vi "Turn_IMU.vi"(0 "Timeout (s)":dbl, 1 "Acceptable Error (Degrees)":dbl, 2 "Target (Degrees)":dbl) -> ()   [LabVIEW 2020]
uses:
  <vilib>/Rock Robotics/WPI/ThirdParty/REV Robotics/REVLib/Typedef/Spark MAX Control Type.ctl
  <vilib>/Rock Robotics/WPI/ThirdParty/Phoenix-LabVIEW/Pigeon IMU/CTRE_PigeonIMU_GetYPR.vi
panel:
  out "Times Target Successful":dbl
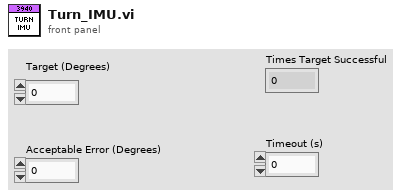
[diagram p1: front panel]
types:
  T1 = typedef "CTRE_PigeonIMU_DeviceRef.ctl" = cluster{"DeviceStatus":errorcluster, "Device Number":u8, "Type":T2, "Device ID":u32, "Handle":u64, "UsageFrame":u32, "Library Path":path}
  T2 = typedef "CTRE_PigeonIMU_ConnectionType.ctl" = u32
  T3 = typedef "WPI_MotorControlDeviceRef.ctl" = cluster{"DeviceStatus":errorcluster, "Type":T4, "PWM":cluster{"PWM Channel":T5, "DeadBand":T6}, "CAN":cluster{"Device Number":u8, "SetOutput VI Ref":variant, "GetOutput VI Ref":variant, "Enable VI Ref":variant, "Disable VI Ref":variant, "Data":variant}, "Invert":bool, "DIO PWM":cluster{"PWM \"Enable\" Channel":T5, "DIOChannel":T7, "PWM Rate":dbl}}
  T4 = typedef "WPI_MotorControlType.ctl" = enum16{"PWM", "CAN", "DIO PWM"}
  T5 = typedef "FPGA_DIOPWMChannel.ctl" = enum8{"PWM 0", "PWM 1", "PWM 2", "PWM 3", "PWM 4", "PWM 5", "PWM 6", "PWM 7", "PWM 8", "PWM 9", "PWM MXP 0", "PWM MXP 1", "PWM MXP 2", "PWM MXP 3", "PWM MXP 4", "PWM MXP 5", "PWM MXP 6", "PWM MXP 7", "PWM MXP 8", "PWM MXP 9", "Invalid"}
  T6 = typedef "WPI_PWMDeadband.ctl" = cluster{"Name":string, "maxPositivePwm":i32, "minPositivePwm":i32, "centerPwm":i32, "maxNegativePwm":i32, "minNegativePwm":i32, "angularRange":u16}
  T7 = typedef "FPGA_DIOChannel.ctl" = enum8{"DIO 0", "DIO 1", "DIO 2", "DIO 3", "DIO 4", "DIO 5", "DIO 6", "DIO 7", "DIO 8", "DIO 9", "DIO MXP 0", "DIO MXP 1", "DIO MXP 2", "DIO MXP 3", "DIO MXP 4", "DIO MXP 5", "DIO MXP 6", "DIO MXP 7", "DIO MXP 8", "DIO MXP 9", "DIO MXP 10", "DIO MXP 11", "DIO MXP 12", "DIO MXP 13", "DIO MXP 14", "DIO MXP 15", "SPI Port CS1", "SPI Port CS2", "SPI Port CS3", "SPI Port MISO", "SPI Port MOSI", "Invalid"}
  T8 = typedef "Spark MAX Control Type.ctl" = enum16{"Percent VBus", "Voltage", "Velocity", "Position", "Smart Motion", "Current", "Smart Velocity"}
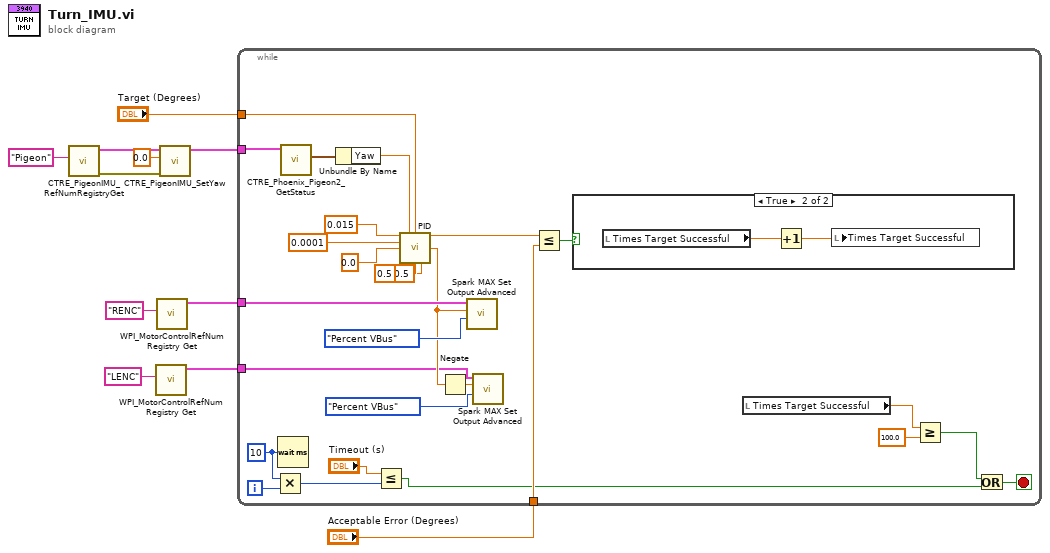
[diagram p0: block diagram]
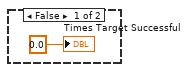
[diagram p2: hidden frame]
diagram:
  n1 = call <vilib>:"CTRE_PigeonIMU_RefNumRegistryGet.vi"("refnum name"="Pigeon") -> ("error out"=w1:errorcluster, "PigeonIMUDevRef"=w4:T1)  [unwired: 9 in]
  n2 = call <vilib>:"WPI_MotorControlRefNum Registry Get.vi"("refnum name"="LENC") -> ("MotorControlDevRef"=w9:T3)  [unwired: 9 in, 1 out]
  n3 = call <vilib>:"WPI_MotorControlRefNum Registry Get.vi"("refnum name"="RENC") -> ("MotorControlDevRef"=w10:T3)  [unwired: 9 in, 1 out]
  n4 = call <vilib>:"CTRE_PigeonIMU_SetYaw.vi"("error in (no error)"=w1, "Value"=0.0, "PigeonIMUDevRef"=w4) -> ("PigeonIMUDevRef"=w3:T1)  [unwired: 7 in, 1 out]
  n5 = while {
    tunnel: w10 -> [w34]
    tunnel: w9 -> [w32]
    tunnel: w3 -> [w30]
    tunnel: "Target (Degrees)" -> [w26]
    tunnel: "Acceptable Error (Degrees)" -> [w24]
    i -> [w20]
    stop <- w16 stop-if-true
    w19 = u32 10 ("milliseconds to wait")
    n6 = Multiply(x=w19, y=w20) -> (x*y=w18:u32)
    n7 = Wait (ms)(milliseconds to wait=w19) -> ()  [unwired: 1 out]
    n8 = call-poly <vilib>:"CTRE_Phoenix_Pigeon2_GetStatus.vi"("PigeonIMUDevRef"=w30) -> ("Yaw Pitch Roll"=w38:cluster{"Yaw":dbl, "Pitch":dbl, "Roll":dbl})  [unwired: 8 in, 2 out]
    n9 = Unbundle By Name(w38) -> ("Yaw"=w35:dbl)
    n10 = Less Or Equal?(x="Timeout (s)", y=w18) -> (x <= y?=w14:bool)
    n11 = call "PID.vi"("Kp"=0.015, "Process Variable"=w35, "Goal"=w26, "Ki"=0.0001, "Kd"=0.0, "Max Ouput"=0.5, "Min Output"=-0.5) -> ("Current Error"=w25:dbl, "Command"=w33:dbl)  [unwired: 6 in, 1 out]
    n12 = Negate(x=w33) -> (-x=w31:dbl)
    n13 = call <vilib>:"Spark MAX Set Output Advanced.vi"("Control Mode"=Spark_MAX_Control_Type."Percent VBus", "Setpoint"=w33, "MotorControlDevRef"=w34) -> ()  [unwired: 7 in, 2 out]
    n14 = call <vilib>:"Spark MAX Set Output Advanced.vi"("Control Mode"=Spark_MAX_Control_Type."Percent VBus", "Setpoint"=w31, "MotorControlDevRef"=w32) -> ()  [unwired: 7 in, 2 out]
    n15 = Less Or Equal?(x=w25, y=w24) -> (x <= y?=w23:bool)
    n16 = case shown="True" w23 {
      frame False {
        "Times Target Successful" <- 0.0
      }
      frame True {
        n17 = local read "Times Target Successful"() -> (w41:dbl)
        n18 = Increment(x=w41) -> (x+1=w40:dbl)
        n19 = local write "Times Target Successful"(w40) -> ()
      }
    }
    n20 = local read "Times Target Successful"() -> (w21:dbl)
    n21 = Greater Or Equal?(x=w21, y=100.0) -> (x >= y?=w15:bool)
    n22 = Or(x=w15, y=w14) -> (x .or. y?=w16:bool)
  }
